vi "Wrap Position.vi"(8 "Position":T1={"Point"={"X col"=0, "Y row"=0}, "Direction"=enum."Up (0x-1y)"}, 9 "New X Col":i32, 10 "New Y Row":i32, 11 "Array":T4[][](array[typedef])) -> (0 "Position Out":T1={"Point"={"X col"=0, "Y row"=0}, "Direction"=enum."Up (0x-1y)"}, 3 "Array Out":T4[][](array[typedef]))   [LabVIEW 2023]
uses:
  Cluster_Position.ctl
  Cluster _Point.ctl
  ENUM_Direction.ctl
  RB ENUM_Board Space ID.ctl
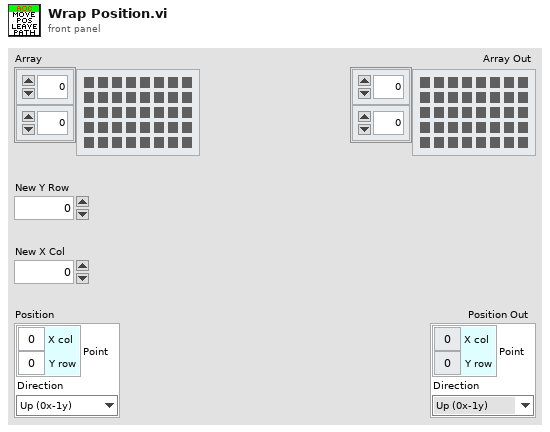
[diagram p1: front panel]
types:
  T1 = typedef "Cluster_Position.ctl" = cluster{"Point":T2, "Direction":T3}
  T2 = typedef "Cluster _Point.ctl" = cluster{"X col":i32, "Y row":i32}
  T3 = typedef "ENUM_Direction.ctl" = enum16{"Right (1x0y)", "Down (0x1y)", "Left (-1x0y)]", "Up (0x-1y)"}
  T4 = typedef "RB ENUM_Board Space ID.ctl" = enum32{"Blank", "Wall", "Tile", "Pos", "path"}
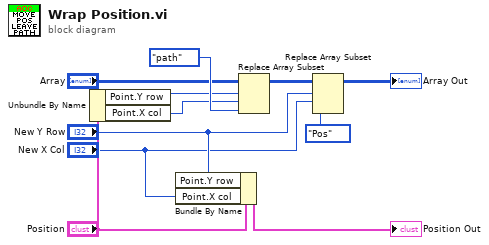
[diagram p0: block diagram]
diagram:
  n1 = Unbundle By Name("Position") -> ("Point.Y row"=w8:i32, "Point.X col"=w9:i32)
  n2 = Bundle By Name(cluster="Position", "Point.Y row"="New Y Row", "Point.X col"="New X Col") -> (→"Position Out":T1)
  n3 = Replace Array Subset(array="Array", new element=RB_ENUM_Board_Space_ID."path" ("new element/subarray"), index (row)=w8, index (col)=w9) -> (w5:T4[][])
  n4 = Replace Array Subset(array=w5, new element=RB_ENUM_Board_Space_ID."Pos" ("new element/subarray"), index (row)="New Y Row", index (col)="New X Col") -> (→"Array Out":T4[][])
